vi "LDA_Cal_Factor_Change.vi"() -> (0 "error out":errorcluster, 4 "Path":path)   [LabVIEW 2012]
panel:
  out "File Changed":bool
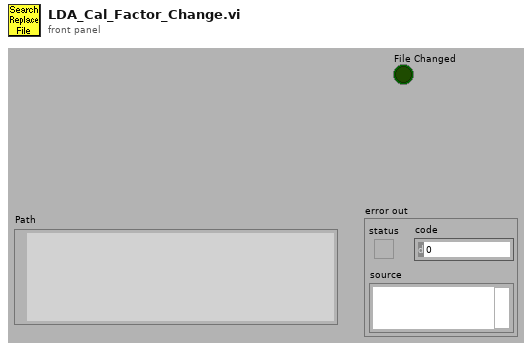
[diagram p1: front panel]
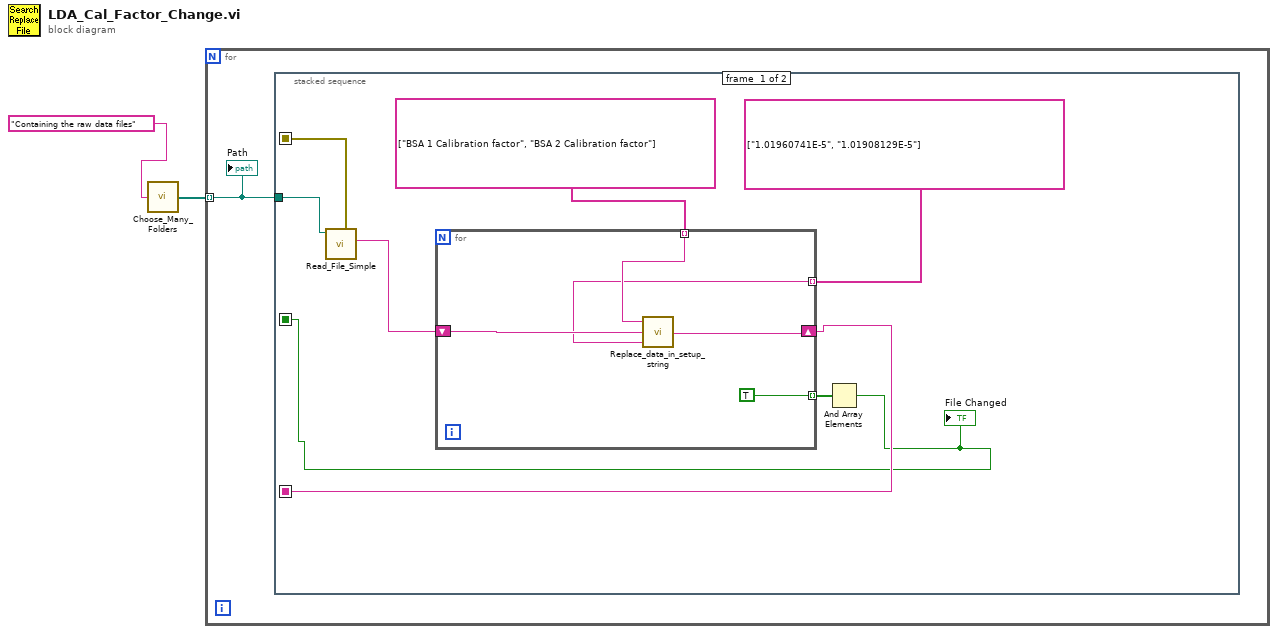
[diagram p0: block diagram]
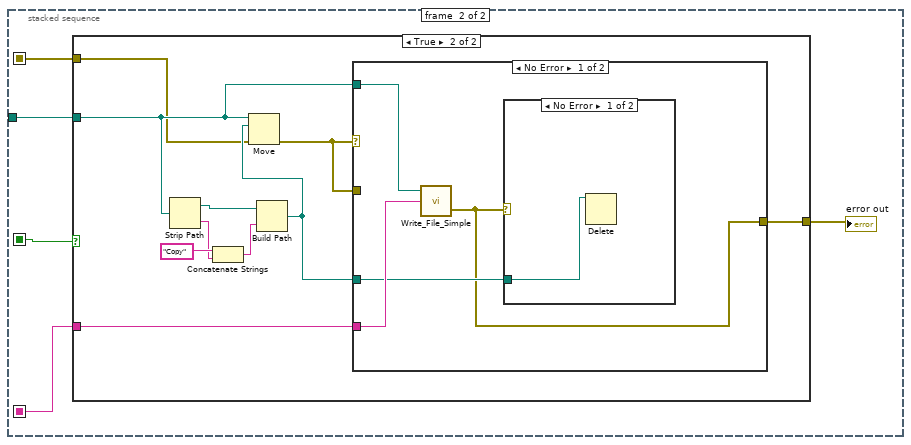
[diagram p2: hidden frame]
diagram:
  n1 = call "Choose_Many_Folders.vi"("Purpose of choosing folder"="Containing the raw data files") -> ("Files"=w1:path[])
  n2 = for {
    tunnel: w1 -> [w3] mode=indexing
    n3 = stacked-sequence {
      seq-local: [w10 _] -> [_ w17]
      seq-local: [w8 _] -> [_ w19]
      seq-local: [w5 _] -> [_ w18]
      tunnel: w3 -> [w11 w21]
      frame #0 {
        n4 = call "Read_File_Simple.vi"("Filename"=w11) -> ("error out"=w10:errorcluster, "string"=w7:string)  [unwired: 4 in, 4 out]
        n5 = for {
          shift-right: [w12] -> w8
          shift-left: w7 -> [w15]
          tunnel: string[] ["BSA 1 Calibration factor", "BSA 2 Calibration factor"] -> [w16] mode=indexing
          tunnel: [TRUE] -> w6 mode=indexing
          tunnel: string[] ["1.01960741E-5", "1.01908129E-5"] -> [w13] mode=indexing
          n6 = call "Replace_data_in_setup_string.vi"("New data string"=w13, "Input string"=w15, "Variable name"=w16) -> ("Appended string"=w12:string)
        }
        n7 = And Array Elements(Boolean array=w6) -> (logical AND=w5:bool)
        "File Changed" <- w5
      }
      frame #1 {
        n8 = case shown="True" w18 {
          tunnel: w21 -> [_ w28]
          tunnel: w19 -> [_ w27]
          tunnel: [w22 w25] -> w20
          tunnel: w17 -> [w22 w23]
          frame False {
          }
          frame True {
            n9 = Strip Path(path=w28) -> (stripped path=w29:path, name=w31:string)
            n10 = Concatenate Strings("Copy" ("name or relative path"), w31) -> (w30:string)
            n11 = Build Path(base path=w29, name or relative path=w30) -> (appended path=w26:path)
            n12 = Move(source path=w28, error in=w23, 10:w26) -> (error out=w24:errorcluster)  [unwired: 2 in, 2 out]
            n13 = case shown="No Error" w24 {
              tunnel: w28 -> [w36 _]
              tunnel: w27 -> [w35 _]
              tunnel: w26 -> [w34 _]
              tunnel: [w33 w38] -> w25
              tunnel: w24 -> [_ w38]
              frame No Error {
                n14 = call "Write_File_Simple.vi"("character string"=w35, "file path"=w36) -> ("error out"=w33:errorcluster)  [unwired: 1 in, 1 out]
                n15 = case shown="No Error" w33 {
                  tunnel: w34 -> [w37 _]
                  frame No Error {
                    n16 = Delete(path (use dialog)=w37) -> ()  [unwired: 4 in, 3 out]
                  }
                  frame Error {
                  }
                }
              }
              frame Error {
              }
            }
          }
        }
        "error out" <- w20
      }
    }
    "Path" <- w3
  }
